vi "power read BAE7.vi"(0 "Max Voltage in":dbl=8.5 format="%.2f", 11 "error in (no error)":errorcluster) -> (4 "normalized Power Read (0-1)":dbl=0.0244140625 format="%.2f", 15 "error out":errorcluster)   [LabVIEW 2014]
doc: "power read BAE7\n\nReads the voltage from an analog input, which serves as a variable for the calculated Normalized power, ranging from 0 -1 V.\n\nNormalized Power = (Vset / Vmax)^2\n\nBeverly Abadines\nPHY 350\nE7"
panel:
  in  "channel (0)":tag="Dev1/ai0"
  # "Power Read BAE7"
  # "Beverly Abadines\nPhys 350\nE7"
  # "Input"
  # "Output"
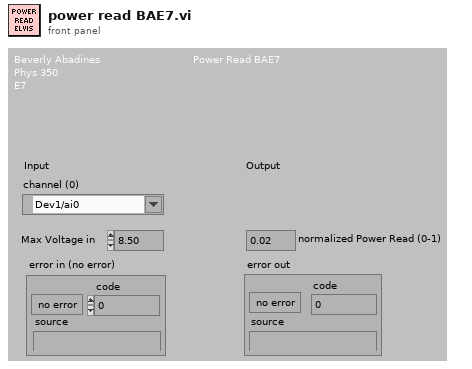
[diagram p1: front panel]
types:
  T1 = enum16{"AI sample channel scan", "AI Waveform triggered"}
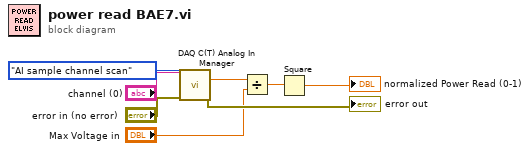
[diagram p0: block diagram]
diagram:
  n1 = call "DAQ C(T) Analog In Manager.vi"("channel (single point) (0)"="channel (0)", "AI mode chooser"=T1."AI sample channel scan", "error in (no error)"="error in (no error)") -> ("V meas"=w4:dbl, "error out"=→"error out":errorcluster)  [unwired: 5 in, 6 out]
  n2 = Divide(x=w4, y="Max Voltage in") -> (x/y=w2:dbl)
  n3 = Square(x=w2) -> (x^2=→"normalized Power Read (0-1)":dbl)
